vi "svx_Timebase TreeInitialize.vi"(8 "State in":T1={"X Scale"={"Name"="Time", "FString"="%#.2g", "Major Color"=16777238, "Minor Color"=16777216, "Grid Style"=1, "Maximum"=0.5, "Minimum"=0.0, "Autoscale"=TRUE, "Show Scale Label"={"Probe X"=FALSE, "Probe Y"=TRUE}, "Show Scale"={"Probe X"=TRUE, "Probe Y"=TRUE}, "Autoscale Once"=FALSE}, "Y Scale"={"Name"="Amplitude", "FString"="%#.2g", "Major Color"=16777238, "Minor Color"=16777216, "Scale Visible"=TRUE, " Label Visible"=TRUE, "Grid Style"=1, "Autoscale"=TRUE, "Maximum"={"Probe X"=1.0, "Probe Y"=1.0}, "Minimum"={"Probe X"=-1.0, "Probe Y"=-1.0}, "Autoscale Once"=FALSE}, "Plot"={"Point Style"=0, "Line Width"=0, "Line Style"=0, "Plot Color"=16860, "Point/fill"=16860}, "Tacho Point Color"=16711680, "Property Name"=[], "Container Bounds"={"Width"=640, "Height"=360}, "Background color"=16777226, "Legend Visible"=TRUE, "Scale Range Change"=refnum, "Strings[]"={"Custom pair name"=FALSE, "Row Strings []"=[], "Column Strings []"=[]}, "Cursor"={"Cursor Point Style"=13, "Cursor Style"=5, "Cursor Line Width"=1, "Cursor Line Style"=0, "Cursor Color"=16860, "Cursor Name Visible"=TRUE, "Cursor Visible"=TRUE, "Cursor Lock"=FALSE, "Cursor Index"=0}, "Index"=[], "Legend Width"=200, " Parents Tags"=[], "Children Tags"=[], "Open?"=[], "Label"="Timebase Plot", "Cursor X Pos"={"X"=0.0, "Y"=0.0}, "Cursor Y Pos"={"X"=0.0, "Y"=0.0}, "Graph Type"=enum."Probe X and Y", "Prev Graph Type"=enum."Probe X and Y", "Prev Legend Visible"=TRUE, "Cursor Release"=refnum, "Pair Strings Changed?"=FALSE, "Cursor ID"=refnum, "Legend Background"=16777226, "Legend Font"=16777222, "Probe Y Label"="Probe Y", "Probe X Label"="Probe X", "Probe X Label Visible"=TRUE, "Probe Y Label Visible"=TRUE, "Tree Item Width"=200, "# Custom RowStr"=0, "# Custom ColStr"=0, "Property Name"=refnum, "Data Related State"=refnum} caption="State", 11 "Tree ref in":refnum<vi>) -> (0 "State out":T1={"X Scale"={"Name"="Time", "FString"="%#.2g", "Major Color"=16777238, "Minor Color"=16777216, "Grid Style"=1, "Maximum"=0.5, "Minimum"=0.0, "Autoscale"=TRUE, "Show Scale Label"={"Probe X"=FALSE, "Probe Y"=TRUE}, "Show Scale"={"Probe X"=TRUE, "Probe Y"=TRUE}, "Autoscale Once"=FALSE}, "Y Scale"={"Name"="Amplitude", "FString"="%#.2g", "Major Color"=16777238, "Minor Color"=16777216, "Scale Visible"=TRUE, " Label Visible"=TRUE, "Grid Style"=1, "Autoscale"=TRUE, "Maximum"={"Probe X"=1.0, "Probe Y"=1.0}, "Minimum"={"Probe X"=-1.0, "Probe Y"=-1.0}, "Autoscale Once"=FALSE}, "Plot"={"Point Style"=0, "Line Width"=0, "Line Style"=0, "Plot Color"=16860, "Point/fill"=16860}, "Tacho Point Color"=16711680, "Property Name"=[], "Container Bounds"={"Width"=640, "Height"=360}, "Background color"=16777226, "Legend Visible"=TRUE, "Scale Range Change"=refnum, "Strings[]"={"Custom pair name"=FALSE, "Row Strings []"=[], "Column Strings []"=[]}, "Cursor"={"Cursor Point Style"=13, "Cursor Style"=5, "Cursor Line Width"=1, "Cursor Line Style"=0, "Cursor Color"=16860, "Cursor Name Visible"=TRUE, "Cursor Visible"=TRUE, "Cursor Lock"=FALSE, "Cursor Index"=0}, "Index"=[], "Legend Width"=200, " Parents Tags"=[], "Children Tags"=[], "Open?"=[], "Label"="Timebase Plot", "Cursor X Pos"={"X"=0.0, "Y"=0.0}, "Cursor Y Pos"={"X"=0.0, "Y"=0.0}, "Graph Type"=enum."Probe X and Y", "Prev Graph Type"=enum."Probe X and Y", "Prev Legend Visible"=TRUE, "Cursor Release"=refnum, "Pair Strings Changed?"=FALSE, "Cursor ID"=refnum, "Legend Background"=16777226, "Legend Font"=16777222, "Probe Y Label"="Probe Y", "Probe X Label"="Probe X", "Probe X Label Visible"=TRUE, "Probe Y Label Visible"=TRUE, "Tree Item Width"=200, "# Custom RowStr"=0, "# Custom ColStr"=0, "Property Name"=refnum, "Data Related State"=refnum} caption="State", 3 "Tree ref out":refnum<vi>)   [LabVIEW 2017, in "SVX Timebase.xctl"]
uses:
  <vilib>/addons/_XControls/Timebase Plot/SVX Timebase.xctl
  <vilib>/addons/_XControls/Timebase Plot/subVIs/svx_Timebase State.ctl
  <vilib>/addons/_XControls/Timebase Plot/subVIs/svx_Timebase Bounds.ctl
  <vilib>/addons/_XControls/Timebase Plot/subVIs/svx_Timebase Graph Types.ctl
  <vilib>/addons/_XControls/Timebase Plot/subVIs/svx_Timebase Data Related State.ctl
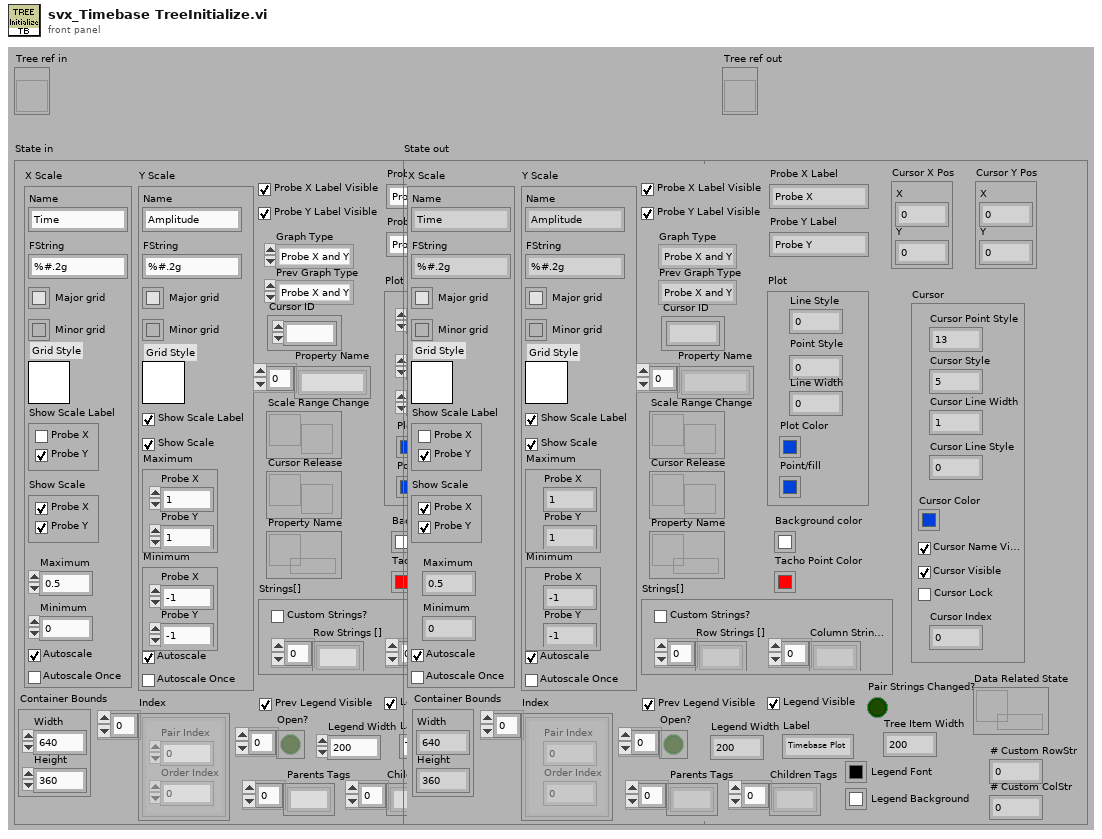
[diagram p1: front panel]
types:
  T1 = typedef "SVX Timebase.xctl/svx_Timebase State.ctl" = cluster{"X Scale":cluster{"Name":string, "FString":string, "Major Color":u32, "Minor Color":u32, "Grid Style":u16, "Maximum":dbl, "Minimum":dbl, "Autoscale":bool, "Show Scale Label":cluster{"Probe X":bool, "Probe Y":bool}, "Show Scale":cluster{"Probe X":bool, "Probe Y":bool}, "Autoscale Once":bool}, "Y Scale":cluster{"Name":string, "FString":string, "Major Color":u32, "Minor Color":u32, "Scale Visible":bool, " Label Visible":bool, "Grid Style":u16, "Autoscale":bool, "Maximum":cluster{"Probe X":dbl, "Probe Y":dbl}, "Minimum":cluster{"Probe X":dbl, "Probe Y":dbl}, "Autoscale Once":bool}, "Plot":cluster{"Point Style":u8, "Line Width":u8, "Line Style":u8, "Plot Color":u32, "Point/fill":u32}, "Tacho Point Color":u32, "Property Name":string[], "Container Bounds":T2, "Background color":u32, "Legend Visible":bool, "Scale Range Change":refnum<user-event>, "Strings[]":cluster{"Custom pair name":bool, "Row Strings []":string[], "Column Strings []":string[]}, "Cursor":cluster{"Cursor Point Style":u8, "Cursor Style":u8, "Cursor Line Width":u8, "Cursor Line Style":u8, "Cursor Color":u32, "Cursor Name Visible":bool, "Cursor Visible":bool, "Cursor Lock":bool, "Cursor Index":i32}, "Index":cluster{"Pair Index":u32, "Order Index":u32}[], "Legend Width":u32, " Parents Tags":string[], "Children Tags":string[], "Open?":bool[], "Label":string, "Cursor X Pos":cluster{"X":dbl, "Y":dbl}, "Cursor Y Pos":cluster{"X":dbl, "Y":dbl}, "Graph Type":T3, "Prev Graph Type":T3, "Prev Legend Visible":bool, "Cursor Release":refnum<user-event>, "Pair Strings Changed?":bool, "Cursor ID":refnum<k1>, "Legend Background":u32, "Legend Font":u32, "Probe Y Label":string, "Probe X Label":string, "Probe X Label Visible":bool, "Probe Y Label Visible":bool, "Tree Item Width":u32, "# Custom RowStr":u32, "# Custom ColStr":u32, "Property Name":refnum<queue>, "Data Related State":T4}
  T2 = typedef "SVX Timebase.xctl/svx_Timebase Bounds.ctl" = cluster{"Width":u32, "Height":u32}
  T3 = typedef "SVX Timebase.xctl/svx_Timebase Graph Types.ctl" = enum16{"Probe X", "Probe Y", "Probe X and Y"}
  T4 = typedef "SVX Timebase.xctl/svx_Timebase Data Related State.ctl" = refnum<queue>
  T5 = enum16{"User-specified Font", "Application Font", "System Font", "Dialog Font"}
  T6 = cluster{"Left Cell String":string, "Child Text":string[], "Child Tag":string, "Item Indent":i32, "Child Only?":bool, "Glyph Index":i32}
  T7 = cluster{"Left Cell String":string, "Child Text":string[], "Child Tag":string, "Item Indent":i32, "Child Only?":bool, "Glyph Index":i32}[]
  T8 = cluster{"left":i16, "top":i16, "right":i16, "bottom":i16}
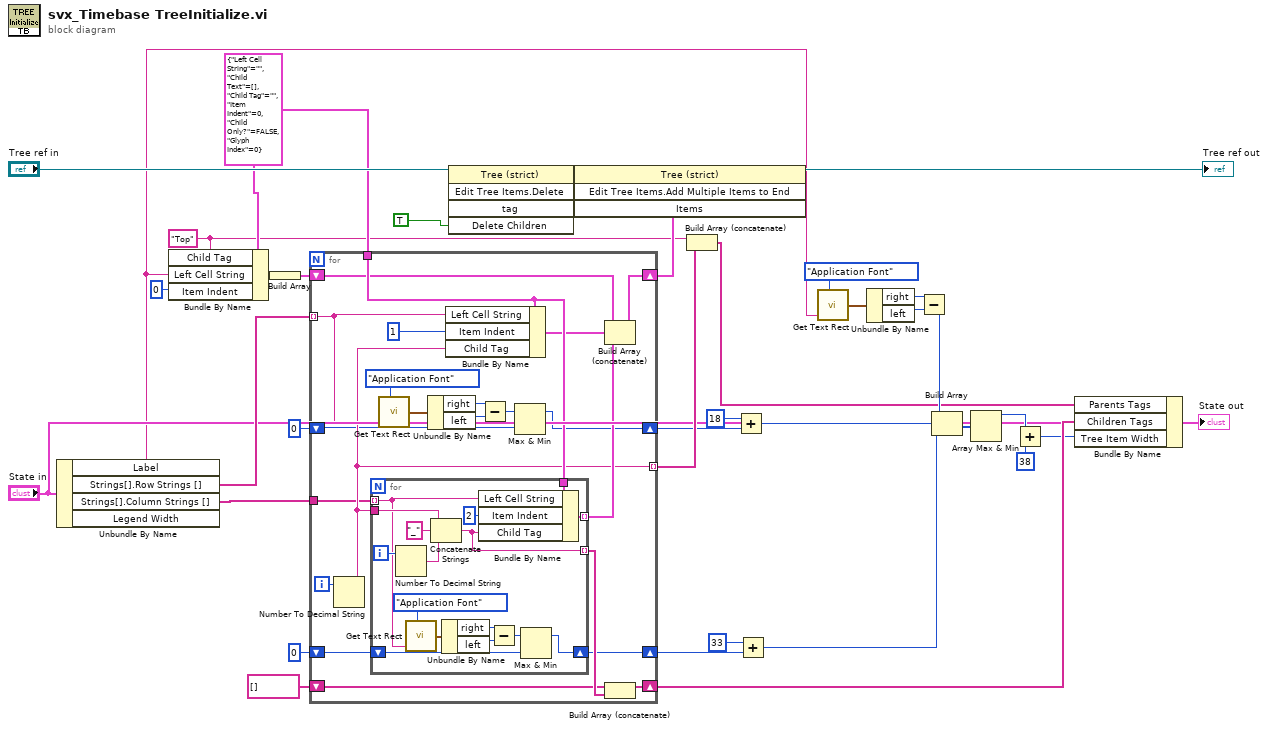
[diagram p0: block diagram]
diagram:
  w26 = "Top" ("Child Tag")
  w33 = T6 {"Left Cell String"="", "Child Text"=[], "Child Tag"="", "Item Indent"=0, "Child Only?"=FALSE, "Glyph Index"=0} ("element")
  n1 = Unbundle By Name("State in") -> ("Label"=w1:string, "Strings[].Row Strings []"=w24:string[], "Strings[].Column Strings []"=w23:string[])  [unwired: 1 out]
  n2 = Bundle By Name(cluster=w33, "Child Tag"=w26, "Left Cell String"=w1, "Item Indent"=0) -> (w32:T6)
  n3 = Build Array(w32) -> (w31:T7)
  n4 = for {
    tunnel: w33 -> [w58]
    tunnel: w24 -> [w40] mode=indexing
    shift-right: [w54] -> w28
    shift-left: w31 -> [w55]
    tunnel: w23 -> [w39]
    shift-right: [w49] -> w4
    shift-left: string[] [] -> [w50]
    tunnel: [w48] -> w25 mode=indexing
    shift-right: [w41] -> w16
    shift-left: i16 0 -> [w42]
    shift-right: [w37] -> w15
    shift-left: i16 0 -> [w38]
    i -> [w52]
    n5 = Number To Decimal String(number=w52) -> (decimal integer string=w48:string)  [unwired: 1 in]
    n6 = for {
      tunnel: w39 -> [w62] mode=indexing
      tunnel: w58 -> [w74]
      tunnel: [w72] -> w53 mode=indexing
      tunnel: [w70] -> w51 mode=indexing
      tunnel: w48 -> [w69]
      shift-right: [w59] -> w37
      shift-left: w38 -> [w60]
      i -> [w68]
      n7 = Number To Decimal String(number=w68) -> (decimal integer string=w67:string)  [unwired: 1 in]
      n8 = call <vilib>:"Get Text Rect.vi"("desired font(Application)"=T5."Application Font", "text"=w62) -> ("rect"=w64:T8)  [unwired: 7 in]
      n9 = Concatenate Strings(w69, "_" ("string"), w67) -> (w70:string)
      n10 = Unbundle By Name(w64) -> ("right"=w65:i16, "left"=w66:i16)
      n11 = Bundle By Name(cluster=w74, "Left Cell String"=w62, "Item Indent"=2, "Child Tag"=w70) -> (w72:T6)
      n12 = Subtract(x=w65, y=w66) -> (x-y=w61:i16)
      n13 = Max & Min(x=w61, y=w60) -> (max(x,y)=w59:i16)  [unwired: 1 out]
    }
    n14 = call <vilib>:"Get Text Rect.vi"("desired font(Application)"=T5."Application Font", "text"=w40) -> ("rect"=w45:T8)  [unwired: 7 in]
    n15 = Unbundle By Name(w45) -> ("right"=w46:i16, "left"=w47:i16)
    n16 = Bundle By Name(cluster=w58, "Left Cell String"=w40, "Item Indent"=1, "Child Tag"=w48) -> (w56:T6)
    n17 = Subtract(x=w46, y=w47) -> (x-y=w43:i16)
    n18 = Max & Min(x=w43, y=w42) -> (max(x,y)=w41:i16)  [unwired: 1 out]
    n19 = Build Array (concatenate)(w55, w56, w53) -> (w54:T7)
    n20 = Build Array (concatenate)(w50, w51) -> (w49:string[])
  }
  n21 = invoke on="Invoke Node" class="Tree (strict)" method="Edit Tree Items.Delete"(reference="Tree ref in", "Delete Children"=TRUE ("Delete Children?")) -> (reference out=w29:refnum<vi>)  [unwired: 3 in, 4 out]
  n22 = invoke on="Invoke Node" class="Tree (strict)" method="Edit Tree Items.Add Multiple Items to End"(reference=w29, "Items"=w28) -> (reference out=→"Tree ref out":refnum<vi>)  [unwired: 2 in, 3 out]
  n23 = Build Array (concatenate)(w26, w25) -> (w5:string[])
  n24 = Add(x=i16 18, y=w16) -> (x+y=w11:i16)
  n25 = Add(x=i16 33, y=w15) -> (x+y=w10:i16)
  n26 = call <vilib>:"Get Text Rect.vi"("desired font(Application)"=T5."Application Font", "text"=w1) -> ("rect"=w21:T8)  [unwired: 7 in]
  n27 = Unbundle By Name(w21) -> ("right"=w20:i16, "left"=w19:i16)
  n28 = Subtract(x=w20, y=w19) -> (x-y=w12:i16)
  n29 = Build Array(w12, w11, w10) -> (w9:i16[])
  n30 = Array Max & Min(array=w9) -> (max value=w7:i16)  [unwired: 3 out]
  n31 = Add(x=w7, y=i16 38) -> (x+y=w3:i16)
  n32 = Bundle By Name(cluster="State in", "Parents Tags"=w5, "Children Tags"=w4, "Tree Item Width"=w3) -> (→"State out":T1)
